vi "Custom Item Symbols-Set Symbol Array.vi"(8 "error in (no error)":errorcluster, 10 "Symbols":T1(array[cluster]), 11 "TreeControl in":refnum<class "TreeControl.lvclass">) -> (0 "error out":errorcluster, 3 "TreeControl out":refnum<class "TreeControl.lvclass">)   [LabVIEW 2015, in "TreeControl.lvclass"]
doc: "Sets the images of all item symbols.\n\n If you want to use a picture to set the symbols, use the Picture to Pixmap VI to convert the data to an <b>image data</b> cluster before using this method. The <b>image</b> clusters you wire to this method are similar to the <b>image data</b> input of the Write JPEG File, Write PNG File, and Write BMP File VIs.\n\n Example\n\nQControl Class wrapper around the <b>TreeControl : Custom Item Symbols:Set To Custom Symbol Array Method</b>.\n<b> </b> <b> </b>\n©2016 Q Software Innovations, LLC (QSI)\nwritten by Quentin Alldredge\nproduced in LabVIEW 2015\n\nsupport@qsoftwareinnovations.com\nwww.qsoftwareinnovations.com\n\nAll rights reserved.\n\nRedistribution and use in source and binary forms, with or without modification, are permitted provided that the following conditions are met:\n\n * Redistributions of source code must retain the above copyright notice, this list of conditions and the following disclaimer.\n * Redistributions in binary form must reproduce the above copyright notice, this list of conditions and the following disclaimer in the documentation and/or other materials provided with the distribution.\n * Neither the name of Q Software Innovations, LLC. nor the names of its contributors may be used to endorse or promote products derived from this software without specific prior written permission.\n\nTHIS SOFTWARE IS PROVIDED BY THE COPYRIGHT HOLDERS AND CONTRIBUTORS \"AS IS\" AND ANY EXPRESS OR IMPLIED WARRANTIES, INCLUDING, BUT NOT LIMITED TO, THE IMPLIED WARRANTIES OF MERCHANTABILITY AND FITNESS FOR A PARTICULAR PURPOSE ARE DISCLAIMED. IN NO EVENT SHALL THE COPYRIGHT OWNER OR CONTRIBUTORS BE LIABLE FOR ANY DIRECT, INDIRECT, INCIDENTAL, SPECIAL, EXEMPLARY, OR CONSEQUENTIAL DAMAGES (INCLUDING, BUT NOT LIMITED TO, PROCUREMENT OF SUBSTITUTE GOODS OR SERVICES; LOSS OF USE, DATA, OR PROFITS; OR BUSINESS INTERRUPTION) HOWEVER CAUSED AND ON ANY THEORY OF LIABILITY, WHETHER IN CONTRACT, STRICT LIABILITY, OR TORT (INCLUDING NEGLIGENCE OR OTHERWISE) ARISING IN ANY WAY OUT OF THE USE OF THIS SOFTWARE, EVEN IF ADVISED OF THE POSSIBILITY OF SUCH DAMAGE."
uses:
  TreeControl.lvclass
  TreeControl.lvclass/TreeControl.ctl
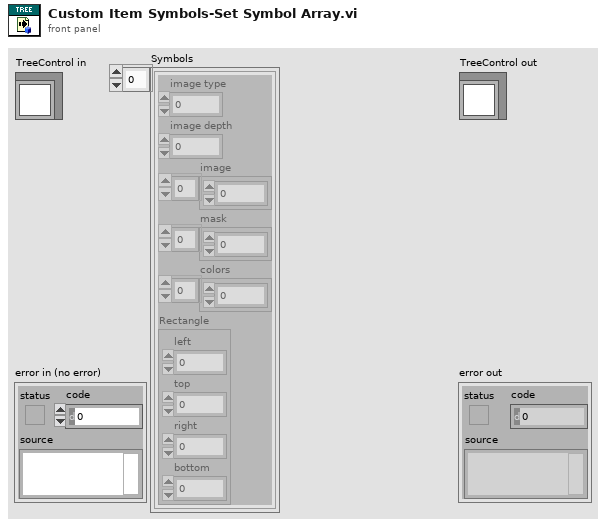
[diagram p1: front panel]
types:
  T1 = cluster{"image type":i32, "image depth":i32, "image":u8[], "mask":u8[], "colors":u32[], "Rectangle":cluster{"left":i16, "top":i16, "right":i16, "bottom":i16}}[]
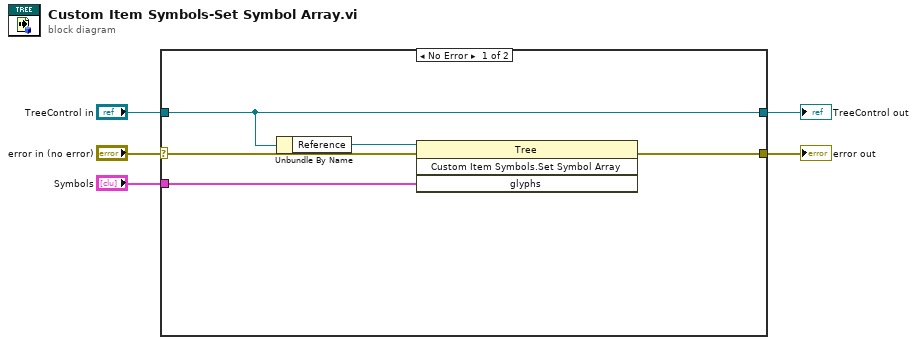
[diagram p0: block diagram]
diagram:
  n1 = case shown="No Error" "error in (no error)" {
    selector: "error in (no error)" -> [w10 w12]
    tunnel: [w9 w12] -> w4
    tunnel: [w8 w11] -> w2
    tunnel: "TreeControl in" -> [w8 w11]
    tunnel: "Symbols" -> [w6 _]
    frame No Error {
      n2 = Unbundle By Name(w8) -> ("Reference"=w7:refnum<vi>)
      n3 = invoke class="Tree" method="Custom Item Symbols.Set Symbol Array"(reference=w7, error in=w10, "glyphs"=w6) -> (error out=w9:errorcluster)  [unwired: 1 in, 3 out]
    }
    frame Error {
    }
  }
  "error out" <- w4
  "TreeControl out" <- w2
